vi "aFGV - Datalog Page.vi"(6 "Action":enum16{"Read", "Write"}(ring)=enum."Write", 8 "Error In":errorcluster, 11 "Data In":T1={"HMI Configuration"={"EXE Name"="", "Project Name"="", "Max Page No"=2, "HMI State"=enum."Invalid", "Version"=enum."Demo", "Check License"=FALSE, "Font Size"=44, "Res: Height"=655, "Res: Width"=1356, "License Level"=enum."Level 2", "License Type"=enum."Perpetual"}, "All HMI Module"=["Module - Alarm Driver.vi", "Module - Alarm Event.vi", "Module - Arduino DIO AI.vi", "Module - DAQmx AI.vi", "Module - DAQmx AO.vi", "Module - DAQmx DI.vi", "Module - DAQmx DO.vi", "Module - Developer.vi", "Module - Error Management.vi", "Module - Login.vi", "Module - P1 Display.vi", "Module - P2 List Device.vi", "Module - P3 Configure Tags IO.vi", "Module - P4 Log Config.vi", "Module - P5 Filter.vi", "Module - P6 Calibration.vi", "Module - P7 Analysis.vi", "Module - P8 User Management.vi", "Module - P9 Favoriot.vi", "Module - P10 Alarm Config.vi"], "Default HMI Module"=["Module - Error Management.vi", "Module - Login.vi", "Module - P1 Display.vi", "Module - P2 List Device.vi", "Module - P3 Configure Tags IO.vi", "Module - P4 Log Config.vi", "Module - P5 Filter.vi", "Module - P6 Calibration.vi", "Module - P7 Analysis.vi", "Module - P8 User Management.vi", "Module - Developer.vi"], "Page Module"=["Module - P1 Display.vi", "Module - P2 List Device.vi", "Module - P3 Configure Tags IO.vi", "Module - P4 Log Config.vi", "Module - P5 Filter.vi", "Module - P6 Calibration.vi", "Module - P8 User Management.vi", "Module - P9 Favoriot.vi"], "Page List: Level 1"=["Module - P1 Display.vi", "Module - P2 List Device.vi", "Module - P3 Configure Tags IO.vi", "Module - P4 Log Config.vi", "Module - P5 Filter.vi", "Module - P6 Calibration.vi", "Module - P8 User Management.vi", "Module - P9 Favoriot.vi"], "Page List: Level 2"=["Module - P1 Display.vi", "Module - P2 List Device.vi", "Module - P3 Configure Tags IO.vi", "Module - P4 Log Config.vi", "Module - P5 Filter.vi", "Module - P6 Calibration.vi"], "Page List: Level 3"=["Module - P1 Display.vi", "Module - P2 List Device.vi", "Module - P3 Configure Tags IO.vi", "Module - P4 Log Config.vi", "Module - P5 Filter.vi", "Module - P6 Calibration.vi", "Module - P8 User Management.vi"], "All RT Module"=[], "Default RT Module"=[], "Acquire Enable Page"=[], "Log Enable Page"=[], "Run Page"=[], "Kill Page"=[], "Button"={"Text"=["MAIN", "DEVICE", "I/O SETTING", "LOGGING", "FILTER", "SCALE", "USER", "CLOUD", "Button 9", "Button 10", "Button 11", "Button 12", "Button 13", "Button 14", "Button 15"], "Tip Strip"=[]}}) -> (0 "Error Out":errorcluster, 3 "Data Out":T1={"HMI Configuration"={"EXE Name"="", "Project Name"="", "Max Page No"=2, "HMI State"=enum."Invalid", "Version"=enum."Demo", "Check License"=FALSE, "Font Size"=44, "Res: Height"=655, "Res: Width"=1356, "License Level"=enum."Level 2", "License Type"=enum."Perpetual"}, "All HMI Module"=["Module - Alarm Driver.vi", "Module - Alarm Event.vi", "Module - Arduino DIO AI.vi", "Module - DAQmx AI.vi", "Module - DAQmx AO.vi", "Module - DAQmx DI.vi", "Module - DAQmx DO.vi", "Module - Developer.vi", "Module - Error Management.vi", "Module - Login.vi", "Module - P1 Display.vi", "Module - P2 List Device.vi", "Module - P3 Configure Tags IO.vi", "Module - P4 Log Config.vi", "Module - P5 Filter.vi", "Module - P6 Calibration.vi", "Module - P7 Analysis.vi", "Module - P8 User Management.vi", "Module - P9 Favoriot.vi", "Module - P9a Alarm Config.vi"], "Default HMI Module"=["Module - Error Management.vi", "Module - Login.vi", "Module - Developer.vi", "Module - P1 Display.vi", "Module - P2 List Device.vi", "Module - P3 Configure Tags IO.vi", "Module - P4 Log Config.vi", "Module - P5 Filter.vi", "Module - P6 Calibration.vi", "Module - P7 Analysis.vi", "Module - P8 User Management.vi", "Module - P9 Favoriot.vi", "Module - P9a Alarm Config.vi", "Module - Alarm Event.vi", "Module - Alarm Driver.vi"], "Page Module"=["Module - P1 Display.vi", "Module - P2 List Device.vi", "Module - P3 Configure Tags IO.vi", "Module - P4 Log Config.vi", "Module - P5 Filter.vi", "Module - P6 Calibration.vi", "Module - P8 User Management.vi", "Module - P9 Favoriot.vi", "Module - P9a Alarm Config.vi"], "Page List: Level 1"=["Module - P1 Display.vi", "Module - P2 List Device.vi", "Module - P3 Configure Tags IO.vi", "Module - P4 Log Config.vi", "Module - P5 Filter.vi", "Module - P6 Calibration.vi", "Module - P8 User Management.vi", "Module - P9 Favoriot.vi", "Module - P9a Alarm Config.vi"], "Page List: Level 2"=["Module - P1 Display.vi", "Module - P2 List Device.vi", "Module - P3 Configure Tags IO.vi", "Module - P4 Log Config.vi", "Module - P5 Filter.vi", "Module - P6 Calibration.vi"], "Page List: Level 3"=["Module - P1 Display.vi", "Module - P2 List Device.vi", "Module - P3 Configure Tags IO.vi", "Module - P4 Log Config.vi", "Module - P5 Filter.vi", "Module - P6 Calibration.vi", "Module - P8 User Management.vi"], "All RT Module"=[], "Default RT Module"=["Module - Login.vi"], "Acquire Enable Page"=[], "Log Enable Page"=[], "Run Page"=["Module - DAQmx AI.vi", "Module - DAQmx AO.vi", "Module - DAQmx DI.vi", "Module - DAQmx DO.vi"], "Kill Page"=["Module - Arduino DIO AI.vi"], "Button"={"Text"=["MAIN", "DEVICE", "I/O SETTING", "LOGGING", "FILTER", "SCALE", "USER", "CLOUD", "ALARM", "Button 10", "Button 11", "Button 12", "Button 13", "Button 14", "Button 15"], "Tip Strip"=[]}})   [LabVIEW 2020]
uses:
  Control/Page List Configuration.ctl
  Control/State - FGV.ctl
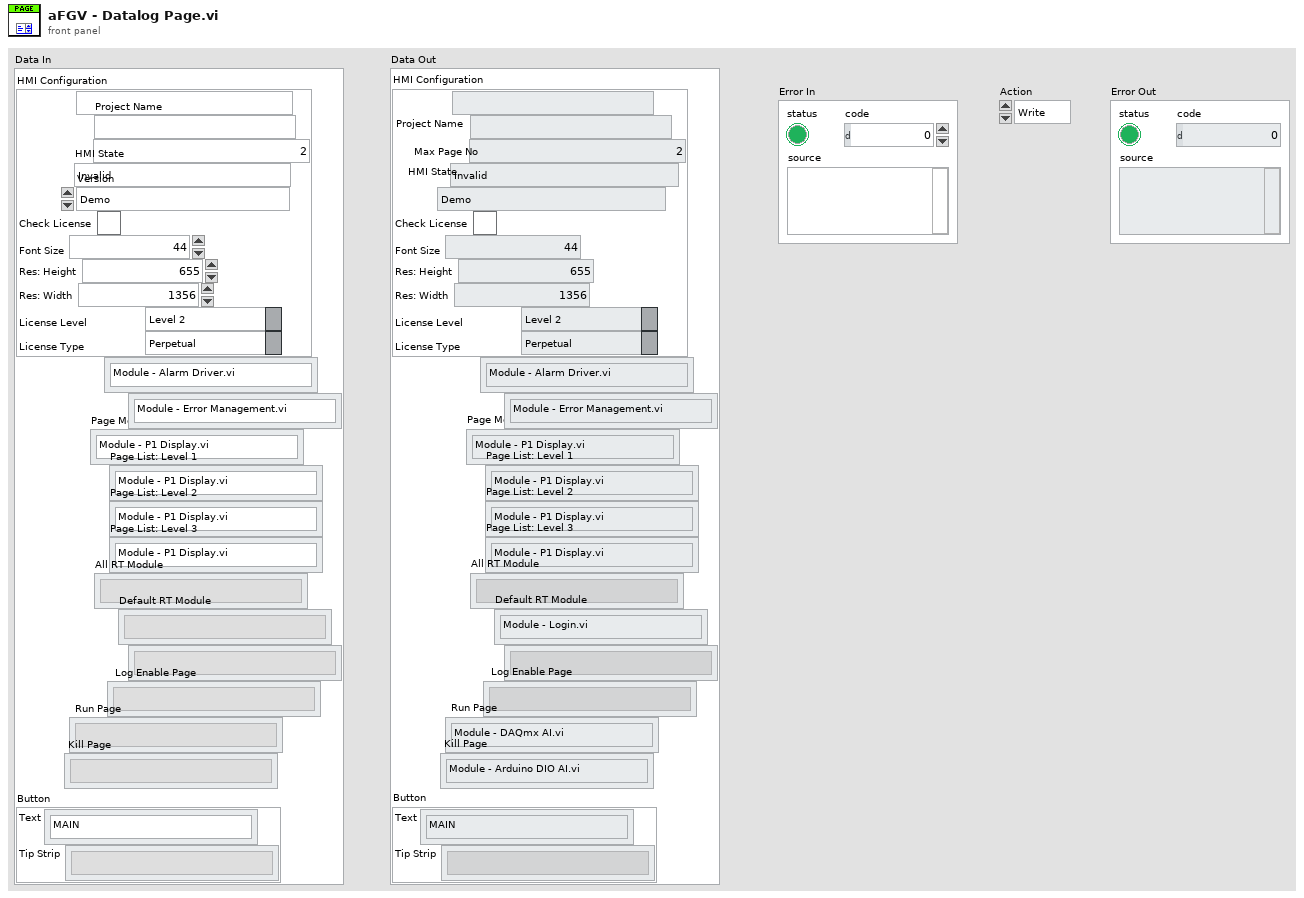
[diagram p1: front panel]
types:
  T1 = typedef "Page List Configuration.ctl" = cluster{"HMI Configuration":cluster{"EXE Name":string, "Project Name":string, "Max Page No":i32, "HMI State":enum32{"Invalid", "Standard", "Closed", "Hidden", "Minimized", "Maximized"}, "Version":enum16{"Demo", "User"}, "Check License":bool, "Font Size":u32, "Res: Height":i16, "Res: Width":i16, "License Level":enum16{"Level 1", "Level 2", "Level 3", "Level 4", "Level 5"}, "License Type":enum16{"Free", "Trial", "Subscription", "Perpetual"}}, "All HMI Module":string[], "Default HMI Module":string[], "Page Module":string[], "Page List: Level 1":string[], "Page List: Level 2":string[], "Page List: Level 3":string[], "All RT Module":string[], "Default RT Module":string[], "Acquire Enable Page":string[], "Log Enable Page":string[], "Run Page":string[], "Kill Page":string[], "Button":cluster{"Text":string[], "Tip Strip":string[]}}
  T2 = typedef "State - FGV.ctl" = enum16{"Write", "Read"}
  T3 = enum16{"open", "replace", "create", "open or create", "replace or create", "replace or create with confirmation"}
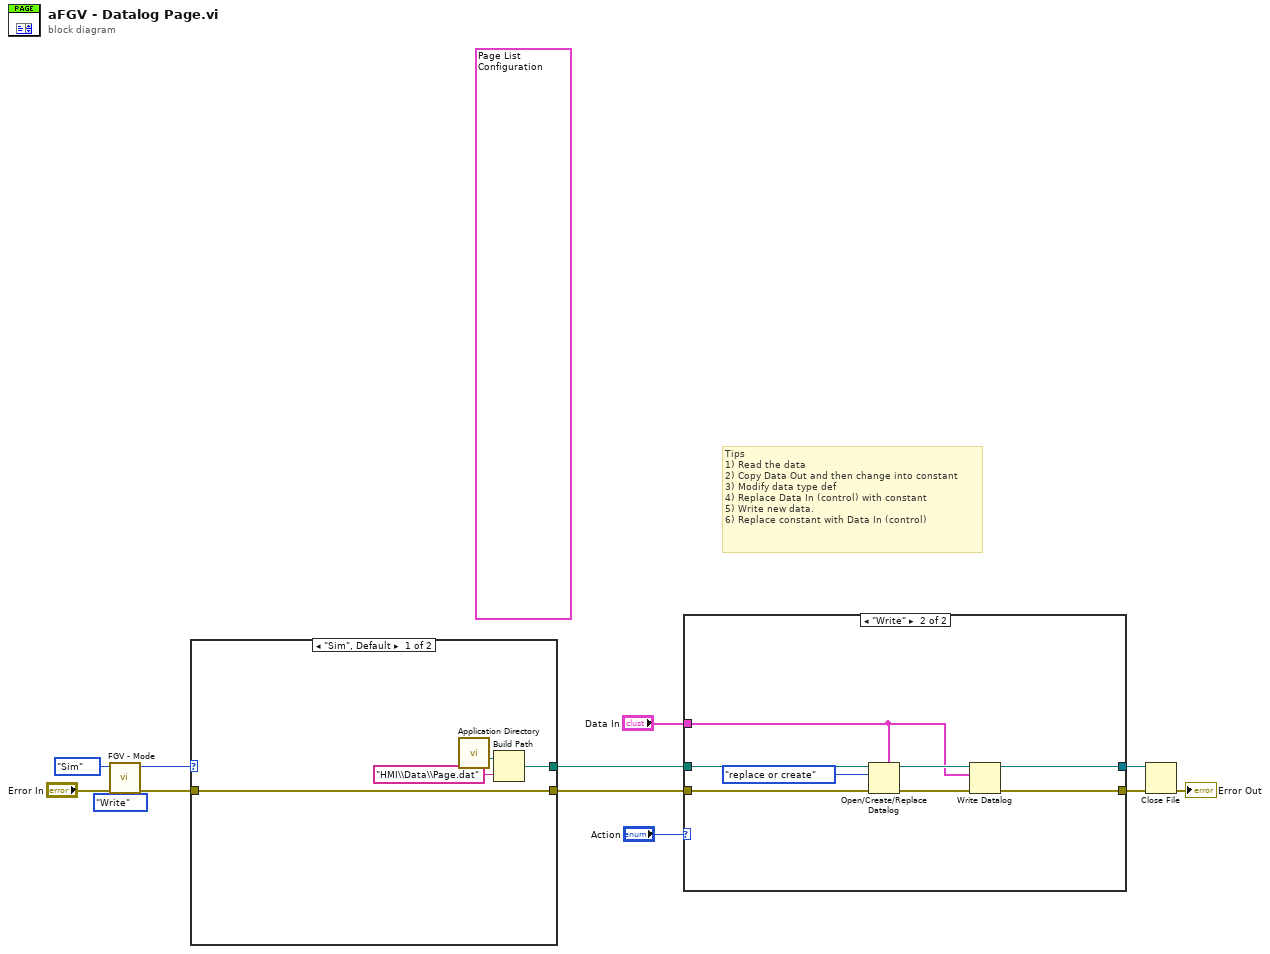
[diagram p0: block diagram]
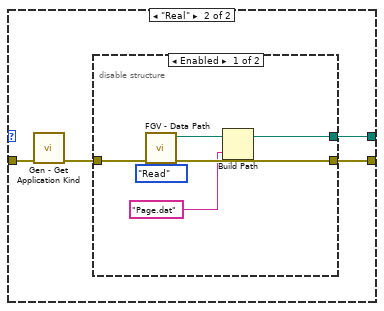
[diagram p2: hidden frame]
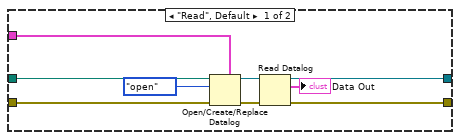
[diagram p4: hidden frame]
diagram:
  (unwired) T1 {"HMI Configuration"={"EXE Name"="VSys Platform", "Project Name"="", "Max Page No"=5, "HMI State"=enum."Maximized", "Version"=enum."User", "Check License"=FALSE, "Font Size"=44, "Res: Height"=655, "Res: Width"=1356, "License Level"=enum."Level 2", "License Type"=enum."Perpetual"}, "All HMI Module"=["Module - Alarm Driver.vi", "Module - Alarm Event.vi", "Module - Analysis.vi", "Module - Arduino DIO AI.vi", "Module - DAQ.vi", "Module - DAQmx AI.vi", "Module - DAQmx AO.vi", "Module - DAQmx DI.vi", "Module - DAQmx DO.vi", "Module - Developer.vi", "Module - Error Management.vi", "Module - License.vi", "Module - Logging.vi", "Module - Login.vi", "Module - Network Stream PC.vi", "Module - NSV Comm PC.vi", "Module - Page Alarm Config.vi", "Module - Page Analysis.vi", "Module - Page Cloud.vi", "Module - Page Configuration.vi", "Module - Page Device.vi", "Module - Page File Transfer.vi", "Module - Page File Viewer.vi", "Module - Page Filter.vi", "Module - Page IO Setting.vi", "Module - Page Main.vi", "Module - Page Prediction.vi", "Module - Page Ranging.vi", "Module - Page Scale.vi", "Module - Page User (Max).vi", "Module - Page User.vi", "Module - Template HMI - Copy.vi", "Module - Template HMI.vi", "Module - WebDAV.vi"], "Default HMI Module"=["Module - Error Management.vi", "Module - Page Main.vi", "Module - Page Prediction.vi", "Module - Page Ranging.vi", "Module - Page User.vi", "Module - Page Configuration.vi", "Module - Login.vi", "Module - Page User (Max).vi"], "Page Module"=["Module - Page Main.vi", "Module - Page Prediction.vi", "Module - Page Ranging.vi", "Module - Page Configuration.vi", "Module - Page User (Max).vi"], "Page List: Level 1"=[], "Page List: Level 2"=[], "Page List: Level 3"=[], "All RT Module"=[], "Default RT Module"=[], "Acquire Enable Page"=[], "Log Enable Page"=[], "Run Page"=[], "Kill Page"=[], "Button"={"Text"=["MAIN", "BUTTON 2", "BUTTON 3", "BUTTON 4", "USER", "BUTTON 6", "BUTTON 7", "BUTTON 8", "BUTTON 9", "BUTTON 10", "BUTTON 11", "BUTTON 12", "BUTTON 13", "BUTTON 14", "BUTTON 15"], "Tip Strip"=["Button 1", "Button 2", "Button 3", "Button 4", "Button 5", "Button 6", "Button 7", "Button 8", "Button 9", "Button 10", "Button 11", "Button 12", "Button 13", "Button 14", "Button 15"]}} ("Data Out 2")
  # "Tips\n1) Read the data\n2) Copy Data Out and then change into constant\n3) Modify data type def\n4) Replace Data In (control) with constant\n5) Write new data.\n6) Replace constant with Data In (control)"
  n1 = call "FGV - Mode.vi"("Action"=enum16{"Read", "Write"}."Write", "Error In"="Error In", "Mode in"=enum16{"Sim", "Real"}."Sim") -> ("Error Out"=w8:errorcluster, "Mode Out"=w4:enum16{"Sim", "Real"})  [unwired: 7 in]
  n2 = case shown="\"Sim\", Default" w4 {
    tunnel: [w16 w20] -> w9
    tunnel: w8 -> [w16 w17]
    tunnel: [w13 w19] -> w2
    frame "Sim", Default {
      n3 = call <vilib>:"Application Directory.vi"() -> ("Application Directory"=w15:path)
      n4 = Build Path(base path=w15, name or relative path="HMI\\Data\\Page.dat") -> (appended path=w13:path)
    }
    frame "Real" {
      n5 = call "Gen - Get Application Kind.vi"("Error In"=w17) -> ("Error Out"=w18:errorcluster)  [unwired: 9 in, 1 out]
      n6 = disable-structure shown="Enabled" {
        disable-tunnel: [w26 w27] -> w20
        disable-tunnel: [w23 _] -> w19
        disable-tunnel: w18 -> [w21 w27]
        frame Enabled {
          n7 = call "FGV - Data Path.vi"("FGV State"=State_-_FGV."Read", "Error In"=w21) -> ("Error Out"=w26:errorcluster, "Path Out"=w25:path)  [unwired: 8 in]
          n8 = Build Path(base path=w25, name or relative path="Page.dat") -> (appended path=w23:path)
        }
        frame Disabled {
        }
      }
    }
  }
  n9 = case shown="\"Write\"" "Action" {
    tunnel: w9 -> [w34 w42]
    tunnel: [w36 w44] -> w12
    tunnel: [w33 w41] -> w7
    tunnel: w2 -> [w32 w40]
    tunnel: "Data In" -> [w30 w37]
    frame "Read", Default {
      n10 = Open/Create/Replace Datalog(5:w30, 8:w34, 10:T3."open" ("operation (0:open)"), 11:w32) -> (0:w35:errorcluster, 3:w31:refnum<k1>)  [unwired: 2 in, 1 out]
      n11 = Read Datalog(4:w35, 7:w31) -> (0:w36:errorcluster, 2:→"Data Out":T1, 3:w33:refnum<k1>)  [unwired: 1 in]
    }
    frame "Write" {
      n12 = Open/Create/Replace Datalog(5:w37, 8:w42, 10:T3."replace or create" ("operation (0:open)"), 11:w40) -> (0:w43:errorcluster, 3:w38:refnum<k1>)  [unwired: 2 in, 1 out]
      n13 = Write Datalog(4:w43, 6:w37, 7:w38) -> (0:w44:errorcluster, 3:w41:refnum<k1>)
    }
  }
  n14 = Close File(refnum=w7, error in=w12) -> (error out=→"Error Out":errorcluster)  [unwired: 1 out]
